vi "BK Precision 983X Series Output ACDC Power.vi"() -> ()   [LabVIEW 2015]
doc: "This example shows how to configure the instrument to output AC+DC power."
uses:
  <instrlib>/BK Precision 983X Series/BK Precision 983X Series.lvlib
panel:
  out "Actual DC Voltage Level (V)":dbl format="%.4g"
  out "Actual DC Current Level (A)":dbl format="%.4g"
  out "Output Frequency (Hz)":dbl format="%.4g"
  out "Actual AC Voltage Level (V)":dbl format="%.4g"
  out "Actual AC Current Level (A)":dbl format="%.4g"
  in  "Output Phase (0.0 degrees)":dbl min=0.0 max=359.7 format="%.1f"
  in  "Output Sync (0: Immediate)":i32(ring) items=["Immediate", "Phase"]
  in  "Frequency (50 Hz)":dbl=50.0 min=43.0 max=1200.0 format="%.3g"
  in  "DC Voltage Level (0.0 V)":dbl format="%.3g"
  in  "AC Voltage Level (0.0 V)":dbl format="%.3g"
  in  "Stop Output":bool
  in  "VISA resource name":refnum<visa-resource-name>
  # "(c) 2017 B&K Precision Corporation.  ALL RIGHTS RESERVED."
  # "degree"
  # "Hz"
  # "V"
  # "V"
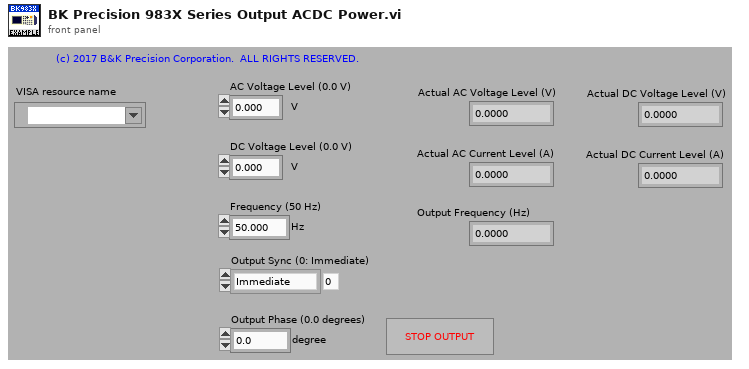
[diagram p1: front panel]
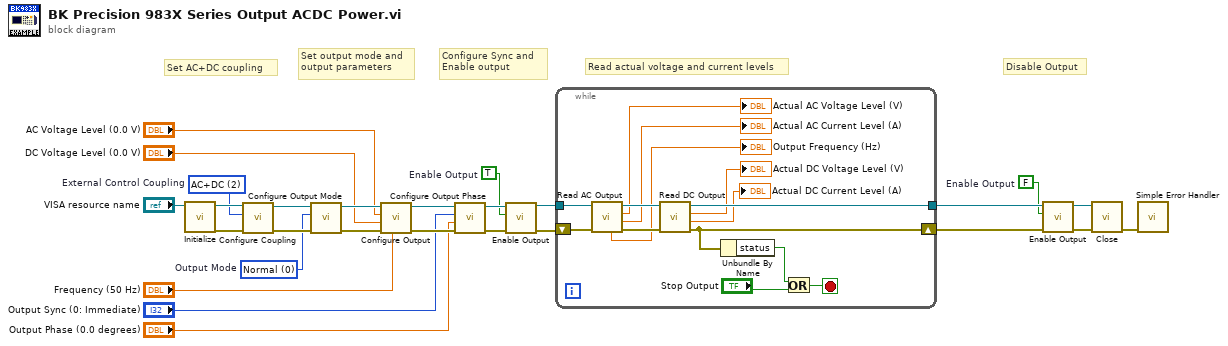
[diagram p0: block diagram]
diagram:
  w20 = u16 0 items=["Normal", "Step", "List", "Pulse"]  # Output Mode
  w23 = u16 2 items=["AC", "DC", "AC+DC"]  # External Control Coupling
  w4 = FALSE  # Enable Output
  w11 = TRUE  # Enable Output
  # "Set output mode and\noutput parameters"
  # "Disable Output"
  # "Read actual voltage and current levels"
  # "Configure Sync and\nEnable output"
  # "Set AC+DC coupling"
  n1 = call <instrlib>:"Initialize.vi"("VISA resource name"="VISA resource name") -> ("error out"=w24:errorcluster, "VISA resource name out"=w25:refnum<visa-resource-name>)  [unwired: 9 in]
  n2 = call <instrlib>:"Configure Coupling.vi"("error in (no error)"=w24, "External Control Coupling (0:AC)"=w23, "VISA resource name"=w25) -> ("error out"=w21:errorcluster, "VISA resource name out"=w22:refnum<visa-resource-name>)  [unwired: 7 in]
  n3 = call <instrlib>:"Configure Output Mode.vi"("error in (no error)"=w21, "Output Mode (0:Normal)"=w20, "VISA resource name"=w22) -> ("error out"=w18:errorcluster, "VISA resource name out"=w19:refnum<visa-resource-name>)  [unwired: 7 in]
  n4 = call <instrlib>:"Configure Output.vi"("Frequency (50 Hz)"="Frequency (50 Hz)", "error in (no error)"=w18, "DC Voltage Level (0.0 V)"="DC Voltage Level (0.0 V)", "AC Voltage Level (0.0 V)"="AC Voltage Level (0.0 V)", "VISA resource name"=w19) -> ("error out"=w17:errorcluster, "VISA resource name out"=w16:refnum<visa-resource-name>)  [unwired: 5 in]
  n5 = call <instrlib>:"Configure Output Phase.vi"("error in (no error)"=w17, "Output Phase (0.0 degrees)"="Output Phase (0.0 degrees)", "Output Sync (0: Immediate)"="Output Sync (0: Immediate)", "VISA resource name"=w16) -> ("error out"=w12:errorcluster, "VISA resource name out"=w13:refnum<visa-resource-name>)  [unwired: 6 in]
  n6 = call <instrlib>:"Enable Output.vi"("error in (no error)"=w12, "Enable Output (F: False)"=w11, "VISA resource name"=w13) -> ("error out"=w10:errorcluster, "VISA resource name out"=w9:refnum<visa-resource-name>)  [unwired: 7 in]
  n7 = while {
    tunnel: [w33] -> w5
    shift-right: [w34] -> w6
    shift-left: w10 -> [w38]
    tunnel: w9 -> [w37]
    stop <- w41 stop-if-true
    n8 = call <instrlib>:"Read AC Output.vi"("error in (no error)"=w38, "VISA resource name"=w37) -> ("error out"=w35:errorcluster, "Actual AC Current Level (A)"=→"Actual AC Current Level (A)":dbl, "Actual AC Voltage Level (V)"=→"Actual AC Voltage Level (V)":dbl, "VISA resource name out"=w36:refnum<visa-resource-name>, "Output Frequency (Hz)"=→"Output Frequency (Hz)":dbl)  [unwired: 5 in]
    n9 = call <instrlib>:"Read DC Output.vi"("error in (no error)"=w35, "VISA resource name"=w36) -> ("error out"=w34:errorcluster, "Actual DC Current Level (A)"=→"Actual DC Current Level (A)":dbl, "Actual DC Voltage Level (V)"=→"Actual DC Voltage Level (V)":dbl, "VISA resource name out"=w33:refnum<visa-resource-name>)  [unwired: 6 in]
    n10 = Unbundle By Name(w34) -> ("status"=w39:bool)
    n11 = Or(x=w39, y="Stop Output") -> (x .or. y?=w41:bool)
  }
  n12 = call <instrlib>:"Enable Output.vi"("error in (no error)"=w6, "Enable Output (F: False)"=w4, "VISA resource name"=w5) -> ("error out"=w7:errorcluster, "VISA resource name out"=w8:refnum<visa-resource-name>)  [unwired: 7 in]
  n13 = call <instrlib>:"Close.vi"("error in (no error)"=w7, "VISA resource name"=w8) -> ("error out"=w26:errorcluster)  [unwired: 9 in]
  n14 = call <vilib>:"Simple Error Handler.vi"("error in (no error)"=w26) -> ()  [unwired: 4 in, 5 out]
